vi "ADAM6060.vi"() -> ()   [LabVIEW 2013]
uses:
  <vilib>/NI Modbus.llb/MB Modbus Command.ctl
panel:
  out "TCP Network Connection Refnum":refnum<k5>
  out "error out":errorcluster
  in  "error in (no error)":errorcluster
  in  "remote port":u16
  in  "address":string
  in  "Discrete":bool[](array[boolean])
  in  "stop":bool
  in  "Modbus Command":T1={"Function Code"=15, "Starting Address"=17, "Quantity"=4, "Data"=[], "Discrete"=[]} {"Function Code" items=["Read Coils"=1, "Read Discrete Inputs"=2, "Read Holding Registers"=3, "Read Input Registers"=4, "Write Single Coil"=5, "Write Single Register"=6, "Read Exception Status"=7, "Write Multiple Coils"=15, "Write Multiple Registers"=16]}
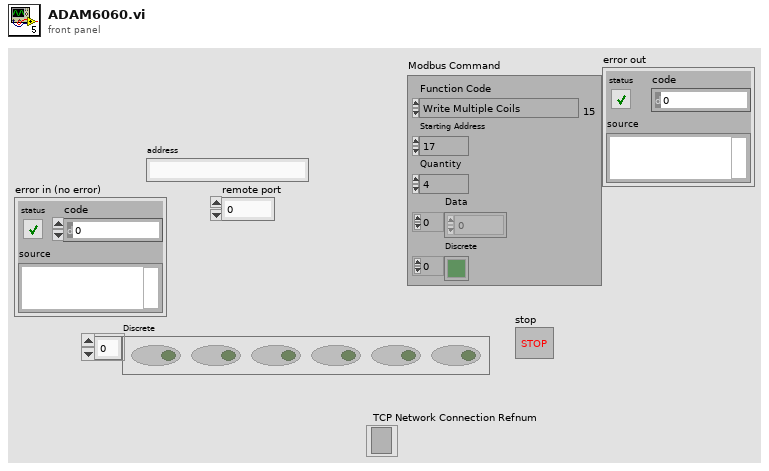
[diagram p1: front panel]
types:
  T1 = typedef "MB Modbus Command.ctl" = cluster{"Function Code":u8, "Starting Address":u16, "Quantity":u16, "Data":u16[], "Discrete":bool[]}
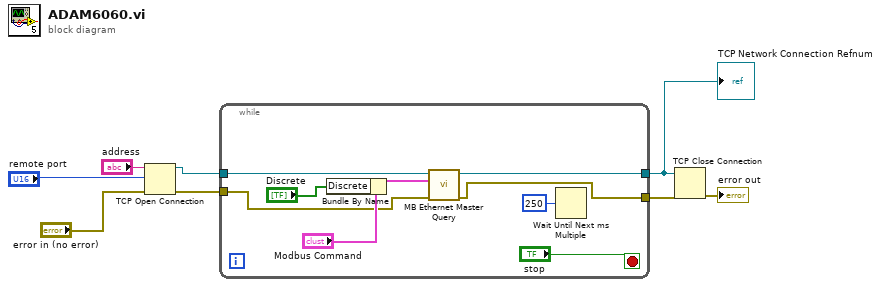
[diagram p0: block diagram]
diagram:
  n1 = TCP Open Connection(address="address", remote port or service name="remote port", error in (no error)="error in (no error)") -> (connection ID=w8:refnum<k5>, error out=w5:errorcluster)  [unwired: 2 in]
  n2 = while {
    tunnel: [w17] -> w1
    tunnel: w8 -> [w16]
    tunnel: w5 -> [w10]
    tunnel: [w9] -> w4
    stop <- "stop" stop-if-true
    n3 = Bundle By Name(cluster="Modbus Command", "Discrete"="Discrete") -> (w15:T1)
    n4 = call <vilib>:"MB Ethernet Master Query.vi"("error in (no error)"=w10, "Modbus Command"=w15, "TCP Connection Refnum in"=w16) -> ("error out"=w9:errorcluster, "TCP Connection Refnum (dup)"=w17:refnum<k5>)  [unwired: 4 in, 3 out]
    n5 = Wait Until Next ms Multiple(millisecond multiple=u32 250) -> ()  [unwired: 1 out]
  }
  "TCP Network Connection Refnum" <- w1
  n6 = TCP Close Connection(connection ID=w1, error in (no error)=w4) -> (error out=→"error out":errorcluster)  [unwired: 1 in, 1 out]
